vi "Read Default Path Cluster.vi"(8 "error in (no error)":errorcluster, 11 "Path Settings in":refnum<class "Path Settings.lvclass">) -> (0 "error out":errorcluster, 2 "Default Path":T1, 3 "Path Settings out":refnum<class "Path Settings.lvclass">)   [LabVIEW 2019, in "Path Settings.lvclass"]
uses:
  Path Settings.lvclass
  Default Path Cluster.ctl
  subVIs/typedefs/Schedule Types/Schedule--Formula.ctl
  Path Settings.lvclass/Path Settings.ctl
  <vilib>/JDP Science/JSONtext/JSONtext.lvlib
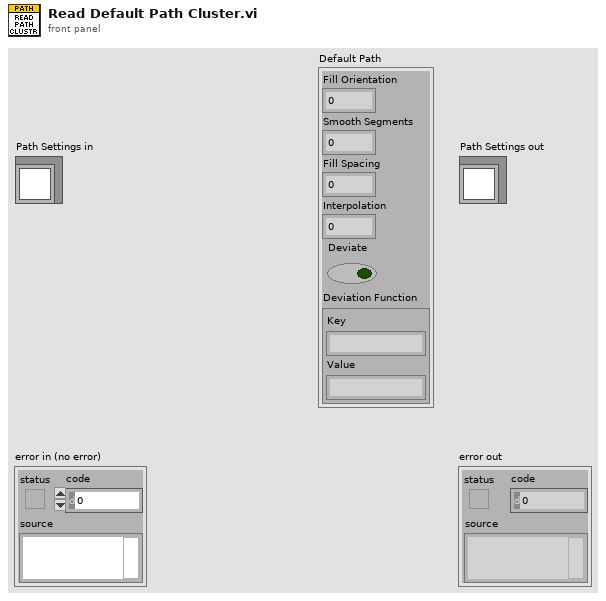
[diagram p1: front panel]
types:
  T1 = typedef "Path Settings.lvclass/Default Path Cluster.ctl" = cluster{"Fill Orientation":u16, "Smooth Segments":dbl, "Fill Spacing":dbl, "Interpolation":dbl, "Deviate":bool, "Deviation Function":cluster{"Key":string, "Value":string}}
  T2 = typedef "Schedule--Formula.ctl" = cluster{"formula":string, "formula length (nm)":dbl, "formula resolution (nm)":dbl}
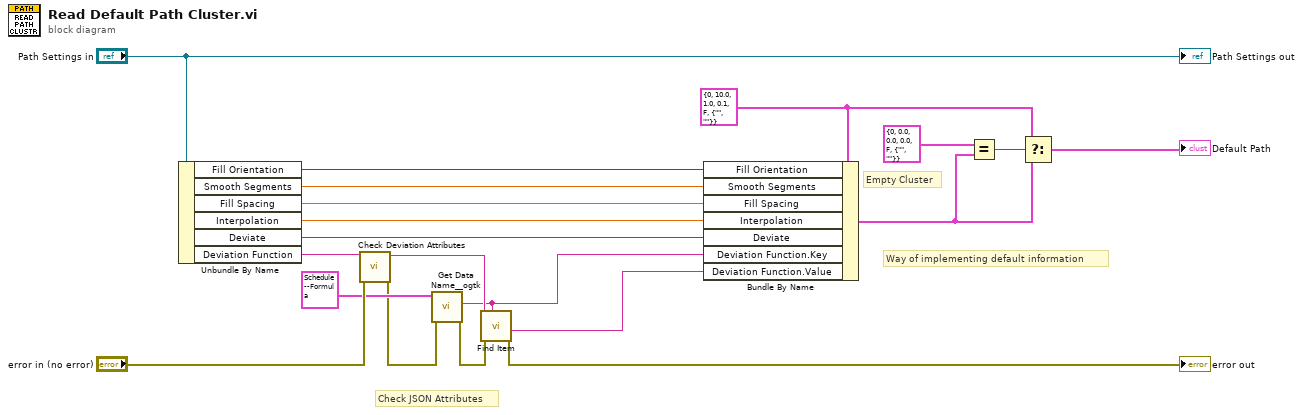
[diagram p0: block diagram]
diagram:
  w14 = T1 {"Fill Orientation"=0, "Smooth Segments"=10.0, "Fill Spacing"=1.0, "Interpolation"=0.1, "Deviate"=FALSE, "Deviation Function"={"Key"="", "Value"=""}} ("cluster")
  # "Check JSON Attributes"
  # "Empty Cluster"
  # "Way of implementing default information"
  n1 = Unbundle By Name("Path Settings in") -> ("Fill Orientation"=w19:u16, "Smooth Segments"=w18:dbl, "Fill Spacing"=w17:dbl, "Interpolation"=w16:dbl, "Deviate"=w10:bool, "Deviation Function"=w9:string)
  n2 = call "Check Deviation Attributes.vi"("error in (no error)"="error in (no error)", "Deviation In"=w9) -> ("error out"=w5:errorcluster, "Deviation Out"=w4:string)  [unwired: 8 in]
  n3 = call <userlib>:"Get Data Name__ogtk.vi"("error in (no error)"=w5, "Data"=T2 {"formula"="1*(step(170-t)*cos(0.62831853071*t)+step(t-170)*cos(0.62831853071*(t-170))*(-1))", "formula length (nm)"=340.0, "formula resolution (nm)"=0.001} ("Formula")) -> ("error out"=w7:errorcluster, "Data Name"=w3:string)  [unwired: 7 in, 1 out]
  n4 = call <vilib>:"Find Item.vi"("$Path or Item Name"=w3, "error in (no error)"=w7, "JSON"=w4) -> ("error out"=→"error out":errorcluster, "<JSON>"=w2:string)  [unwired: 5 in, 2 out]
  n5 = Bundle By Name(cluster=w14, "Fill Orientation"=w19, "Smooth Segments"=w18, "Fill Spacing"=w17, "Interpolation"=w16, "Deviate"=w10, "Deviation Function.Key"=w3, "Deviation Function.Value"=w2) -> (w12:T1)
  n6 = Equal?(x=T1 {"Fill Orientation"=0, "Smooth Segments"=0.0, "Fill Spacing"=0.0, "Interpolation"=0.0, "Deviate"=FALSE, "Deviation Function"={"Key"="", "Value"=""}} ("output cluster"), y=w12) -> (x = y?=w13:bool)
  n7 = Select(t=w14, s=w13, f=w12) -> (s? t:f=→"Default Path":T1)
  "Path Settings out" <- "Path Settings in"
